vi "DOConfigureIdle.vi"(0 "object in":refnum<class "AD2_DO_SDK.lvclass">, 2 "DOSingleCh":T1 {"IdleState" items=["PushPull", "OpenDrain", "OpenSource", "TriState"]; "DigitalOutOutput" items=["Pulse", "Custom", "Random"]; "Type" items=["Pulse", "Custom", "Random"]}, 5 "error in (no error)":errorcluster) -> (14 "object out":refnum<class "AD2_DO_SDK.lvclass">, 16 "DOSingleCh":T1 {"IdleState" items=["PushPull", "OpenDrain", "OpenSource", "TriState"]; "DigitalOutOutput" items=["Pulse", "Custom", "Random"]; "Type" items=["Pulse", "Custom", "Random"]}, 19 "error out":errorcluster)   [LabVIEW 2021, in "AD2_DO_SDK.lvclass"]
uses:
  AD2_DO_SDK.lvclass
  DOSingleCh.ctl
  AD2_DO_SDK.lvclass/AD2_DO_SDK.ctl
  Olasdwf/Olasdwf.lvlib
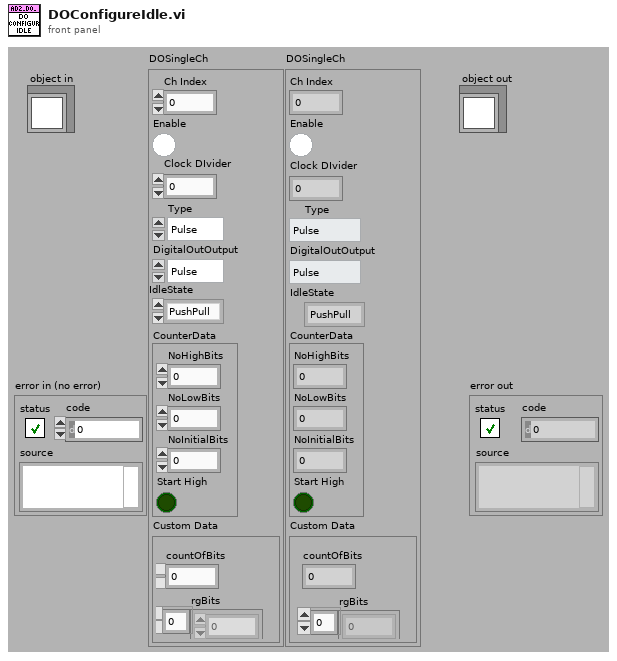
[diagram p1: front panel]
types:
  T1 = typedef "AD2_DO_SDK.lvclass/DOSingleCh.ctl" = cluster{"Ch Index":i32, "Enable":bool, "Clock DIvider":u32, "Type":i32, "DigitalOutOutput":u16, "IdleState":u16, "CounterData":cluster{"NoHighBits":u32, "NoLowBits":u32, "NoInitialBits":u32, "Start High":bool}, "Custom Data":cluster{"countOfBits":u32, "rgBits":u8[]}}
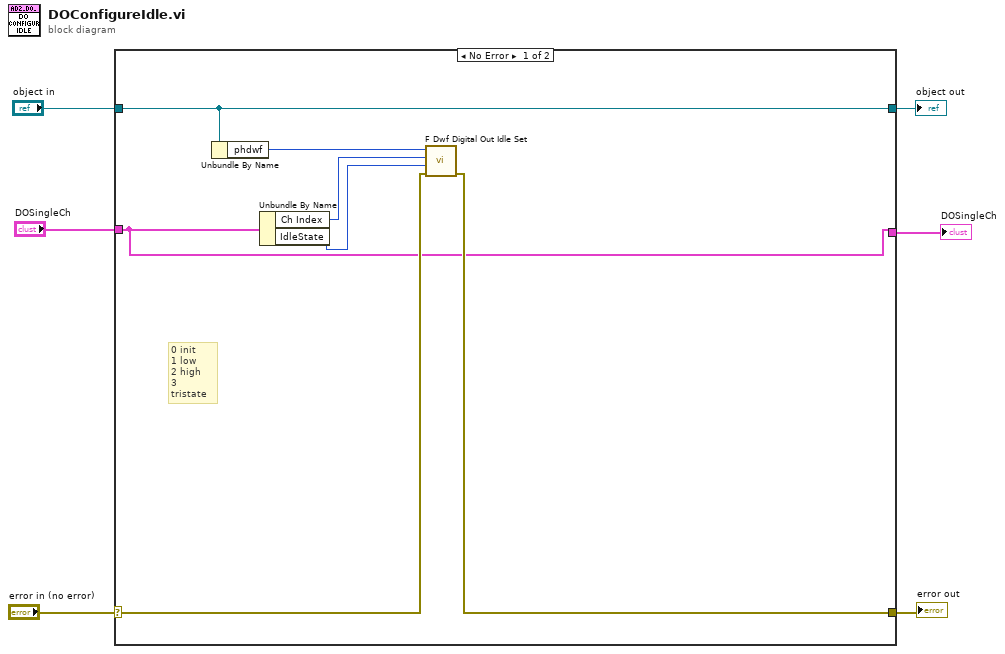
[diagram p0: block diagram]
diagram:
  n1 = case shown="No Error" "error in (no error)" {
    selector: "error in (no error)" -> [w9 w16]
    tunnel: [w8 w16] -> w5
    tunnel: [w13 w15] -> w3
    tunnel: "object in" -> [w13 w15]
    tunnel: "DOSingleCh" -> [w7 w14]
    tunnel: [w7 w14] -> w1
    frame No Error {
      # "0 init\n1 low\n2 high\n3 tristate"
      n2 = Unbundle By Name(w13) -> ("phdwf"=w12:i32)
      n3 = Unbundle By Name(w7) -> ("Ch Index"=w11:i32, "IdleState"=w10:u16)
      n4 = call "F Dwf Digital Out Idle Set.vi"("error in (no error)"=w9, "v"=w10, "idxChannel"=w11, "hdwf"=w12) -> ("error out"=w8:errorcluster)  [unwired: 6 in, 1 out]
    }
    frame Error {
    }
  }
  "error out" <- w5
  "object out" <- w3
  "DOSingleCh" <- w1
